vi "Get Default Data From Variant.vi"() -> ()   [LabVIEW 2012, in "TD Tools.lvlib"]
uses:
  TD Tools.lvlib
panel:
  out "错误输出":errorcluster
  in  "错误输入":errorcluster
  out "Default VData":variant
  in  "Variant":variant
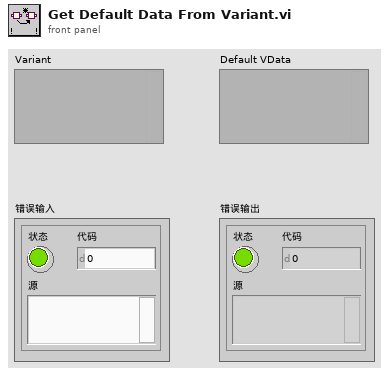
[diagram p1: front panel]
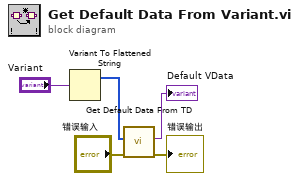
[diagram p0: block diagram]
diagram:
  n1 = Variant To Flattened String(Variant="Variant") -> (1:w4:i16[])  [unwired: 1 out]
  n2 = call "Get Default Data From TD.vi"("错误输入"="错误输入", "Type Descriptor"=w4) -> ("错误输出"=→"错误输出":errorcluster, "Default VData"=→"Default VData":variant)  [unwired: 8 in]
